vi "主界面.vi"() -> ()   [LabVIEW 2010]
uses:
  全局量/试验配置信息.vi
  全局量/全局_配置.vi
  全局量/自动测试结果.vi
panel:
  in  "进度提示":string
  in  "加载配置文件列表":u16(ring)
  out "配置文件路径":path
  out "配置文件目录":path
  in  "通道及参数配置":bool
  in  "?":enum32{"板卡类型1", "板卡类型2"}(tab)
  in  "单选_数字量输入":bool
  in  "单选_数字量输出":bool
  in  "单选_DSP输入":bool
  in  "单选_CAN检测":bool
  in  "单选_LAN检测":bool
  in  "单选_R232检测":bool
  in  "btn_数字输出":bool
  in  "btn_DSP输入":bool
  in  "btn_CAN总线":bool
  in  "btn_LAN总线":bool
  in  "btn_R232_485总线":bool
  in  "btn_开始检测":bool
  in  "btn_数字输入":bool
  in  "单选_R485检测":bool
  in  "单选_AD输入":bool
  out "数字量输入检测":bool
  out "数字量输出检测":bool
  out "模拟量DSP输入检测":bool
  out "模拟量AD输入检测":bool
  out "CAN总线检测":bool
  out "LAN总线检测":bool
  out "RS232总线检测":bool
  out "RS485总线检测":bool
  in  "btn_自动开始检测类型2":bool
  in  "函数类型 4":bool caption="y =f4(A1sin(2*π*A2)x+A3)"
  in  "函数类型 3":bool caption="y =f3(x)"
  in  "函数类型 2":bool caption="y =f2(x,A1,A2,t)"
  in  "函数类型 1":bool caption="y =f1(A1*x+A2)"
  out "函数类型4检测":bool
  out "函数类型3检测":bool
  out "函数类型2检测":bool
  out "函数类型1检测":bool
  in  "单选_函数类型4":bool
  in  "单选_函数类型3":bool
  in  "单选_函数类型2":bool
  in  "单选_函数类型1":bool
  in  "进度每次增加数":dbl
  in  "btn_二维码识别":bool
  out "退出？":bool
  in  "btn_退出":bool
  in  "btn_报告管理":bool
  in  "str_测试地点":string
  in  "str_测试人员":string
  in  "str_测试编号":string
  in  "str_报告编号":string
  # "板卡综合测试装置"
  # "板 卡 测 试 信 息"
  # "试验报告编号："
  # "测试板卡编号："
  # "板卡类型："
  # "测试人员："
  # "测试地点："
  # "自动测试"
  # "分步测试"
  # "测试\n项\n目"
  # "分步测试"
  # "自动测试"
  # "测试\n项\n目"
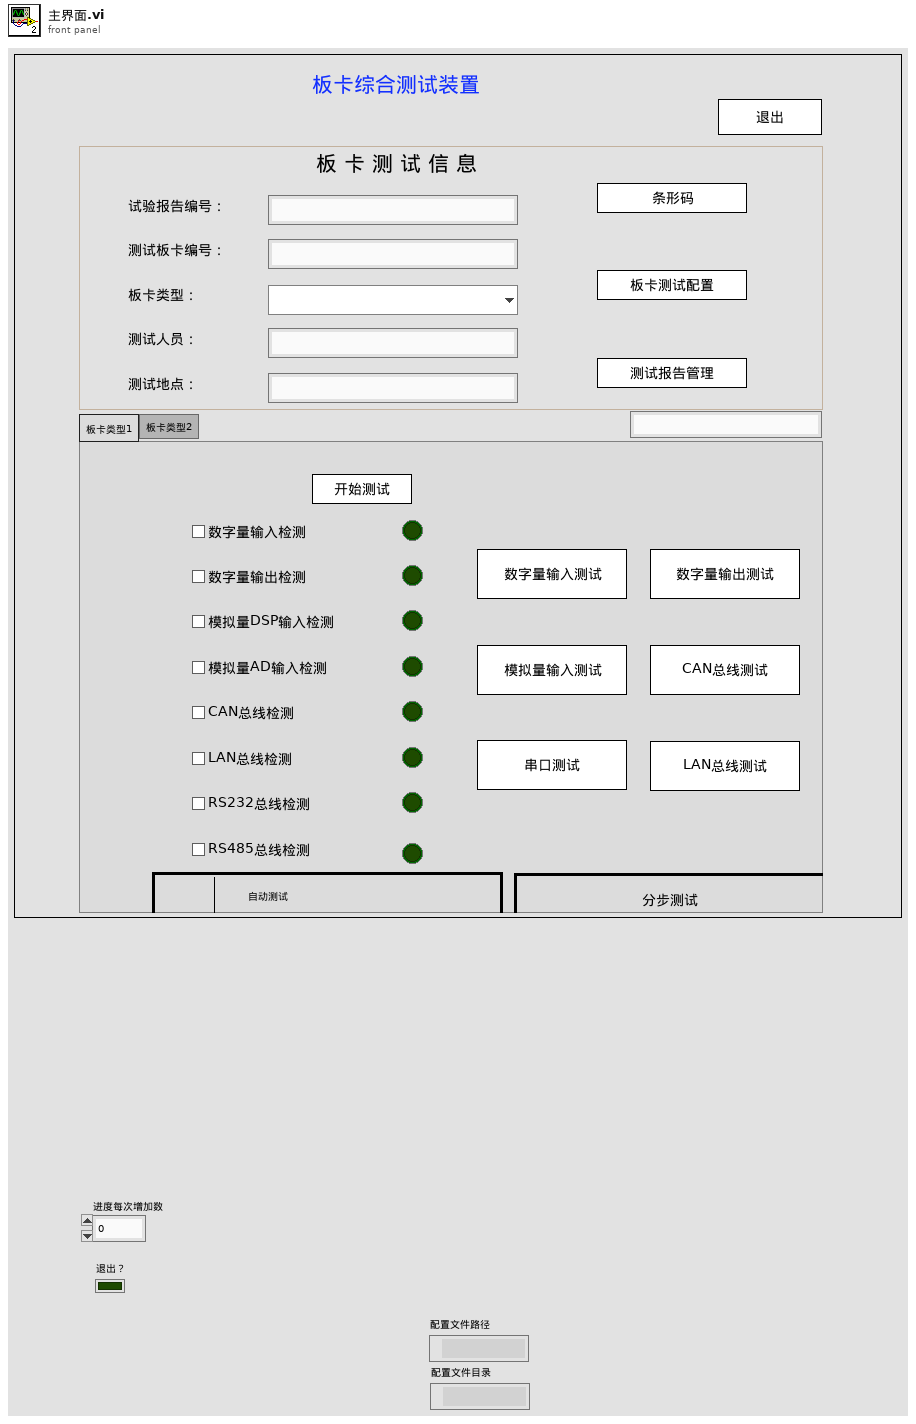
[diagram p1: front panel]
types:
  T1 = cluster{"str_报告编号":string, "str_测试编号":string, "RingText.Text":string, "str_测试人员":string, "str_测试地点":string}
  T2 = enum8{"Enabled", "Disabled", "Disabled and Grayed Out"}
  T3 = cluster{"数字量输入信号路数":i32, "数字量输出信号路数":i32, "DSP模拟量输入信号路数":u32, "DSP模拟量输入信号幅值":u32, "AD模拟量输入信号路数":u32, "AD模拟量输入信号幅值":u32, "RS232端口":u32, "RS232通信路数":u32, "RS232波特率":dbl, "RS485端口":u32, "RS485通信路数":u32, "RS485波特率":u32, "CAN通信路数":i32, "CAN波特率":u32, "以太网选择?":bool, "控制板IP":string, "以太网端口":u32}
  T4 = cluster{"str_报告编号":string, "str_测试编号":string, "RingText.Text":string, "str_测试地点":string, "str_测试人员":string}
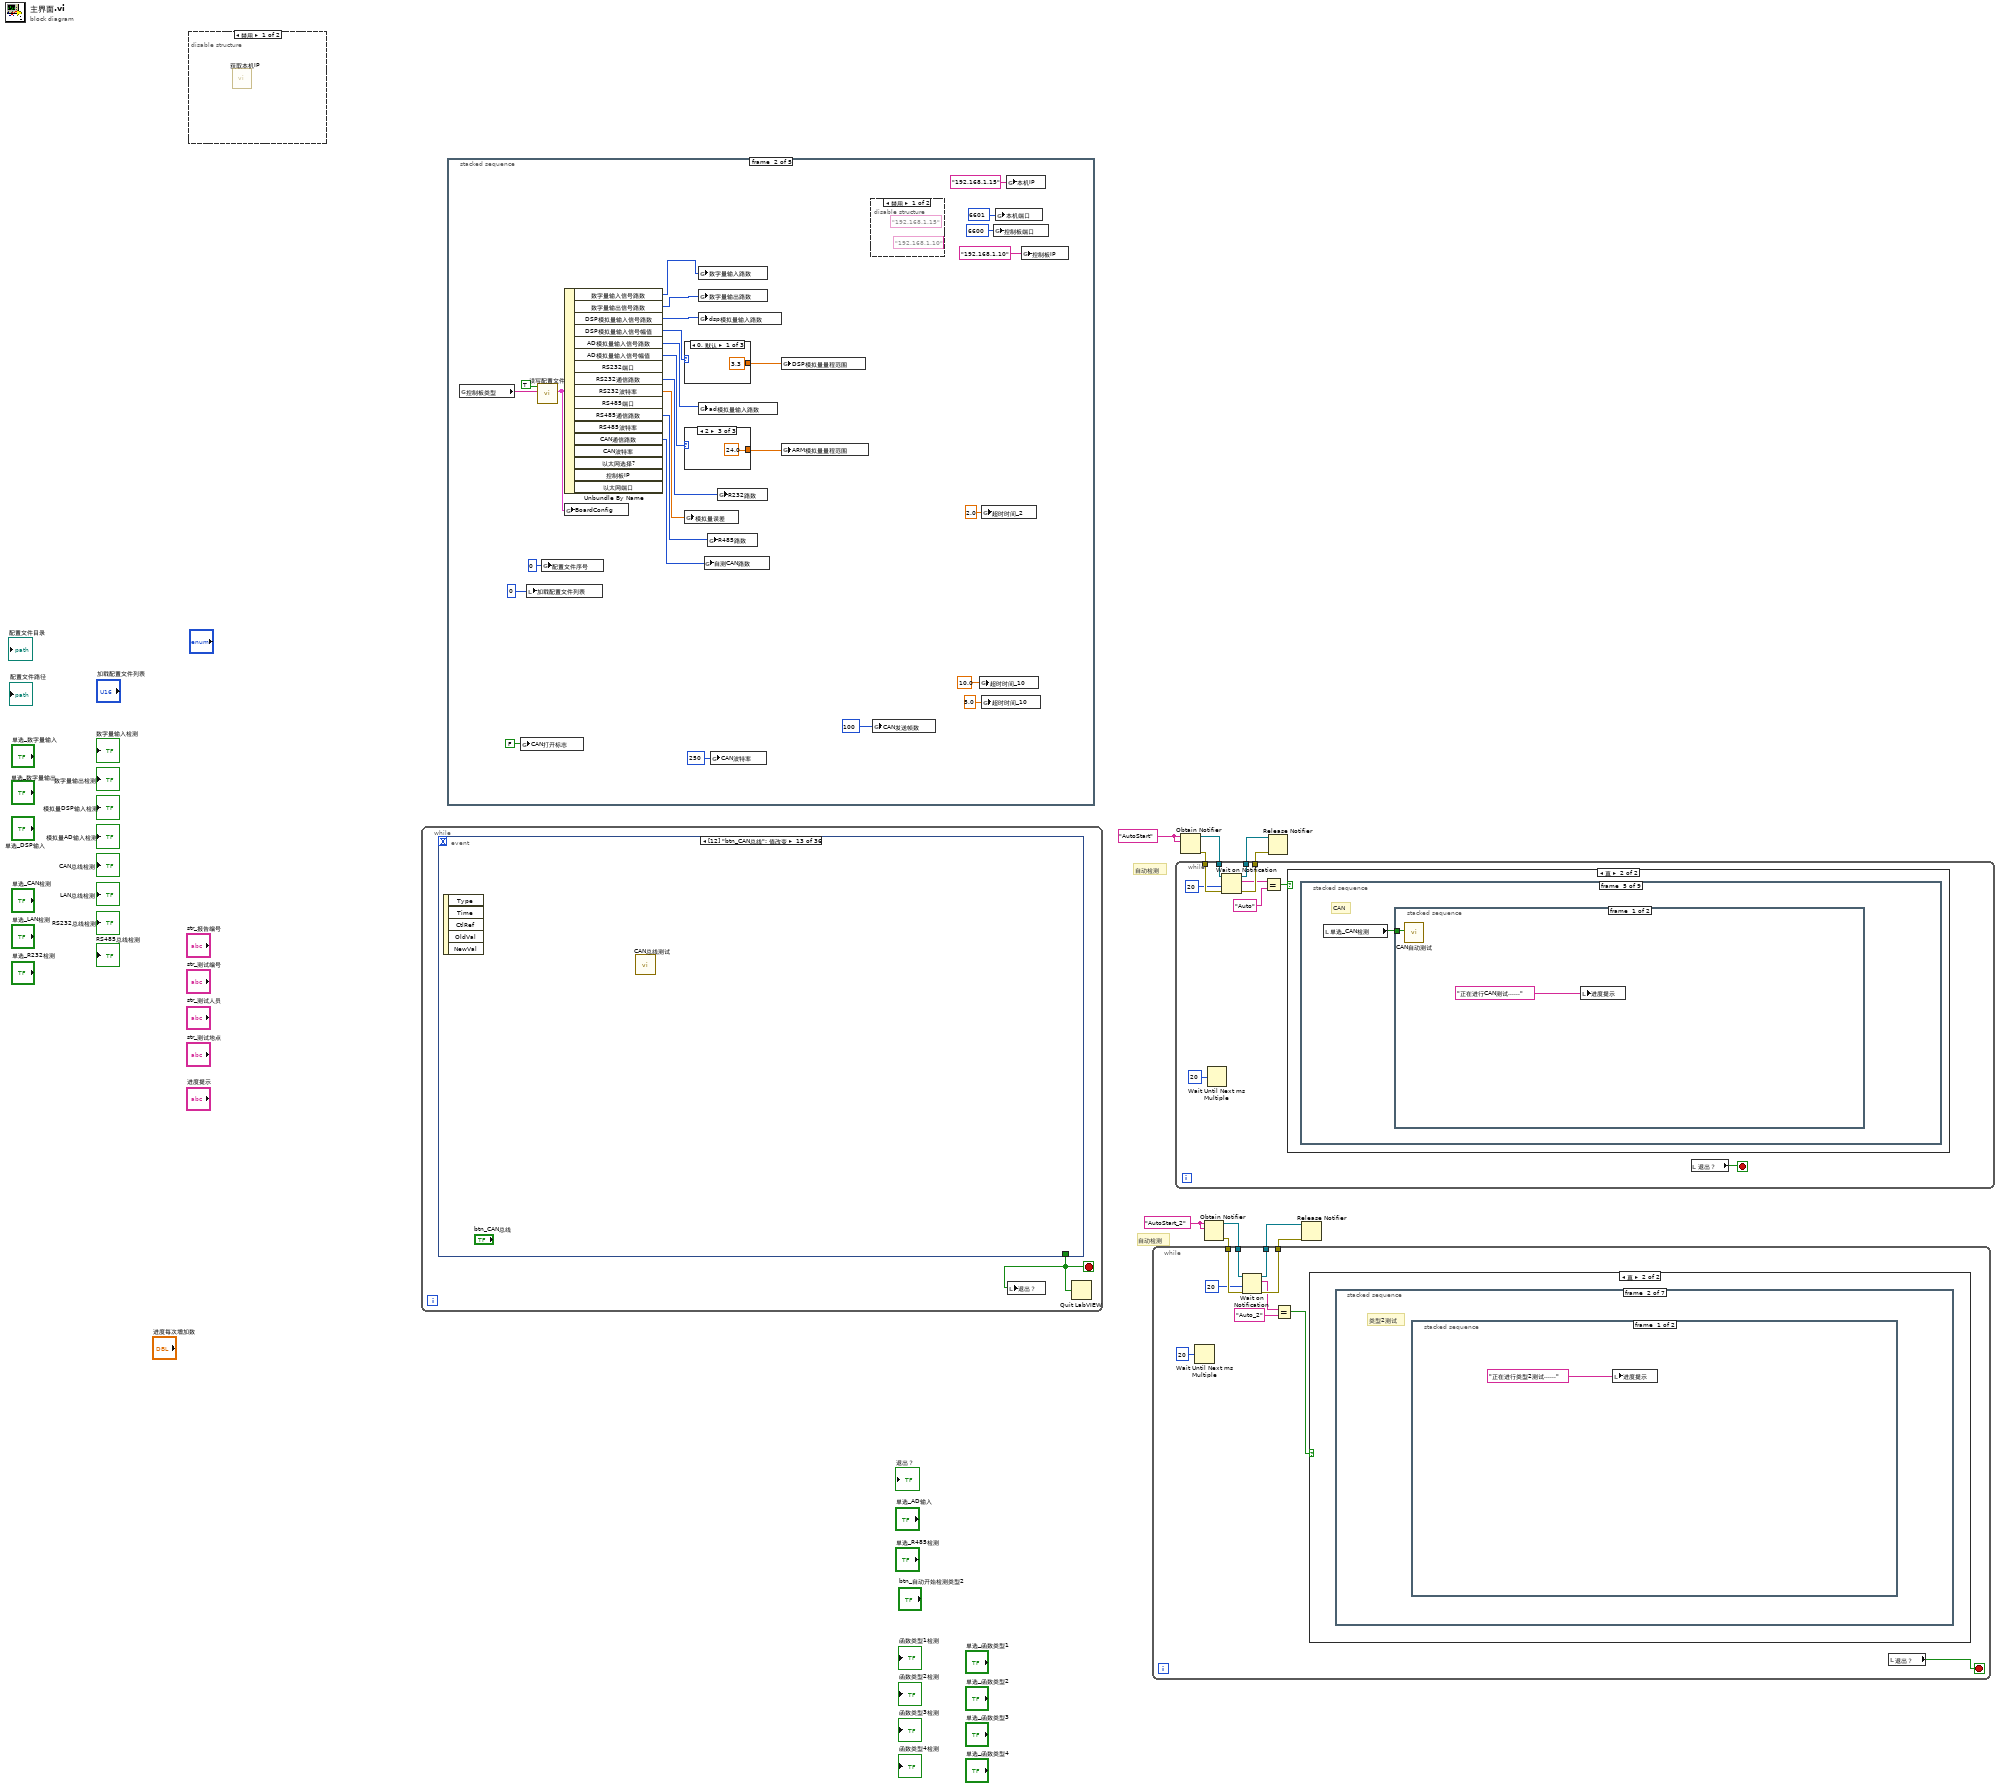
[diagram p0: block diagram]
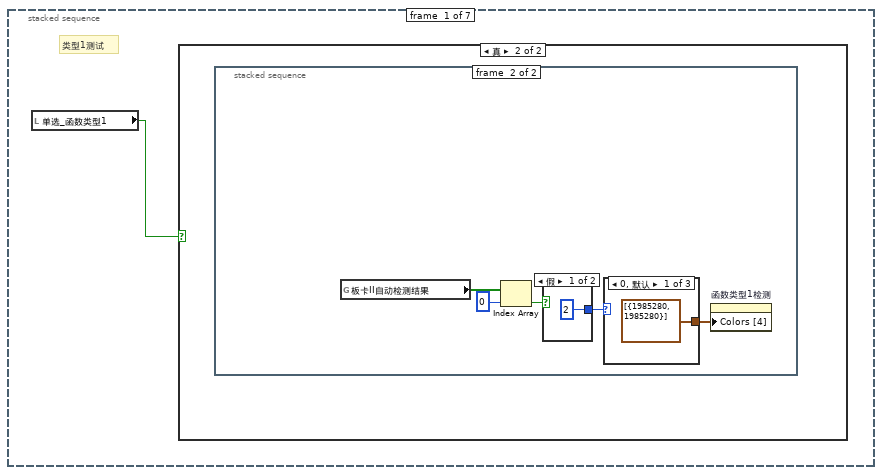
[diagram p4: hidden frame]
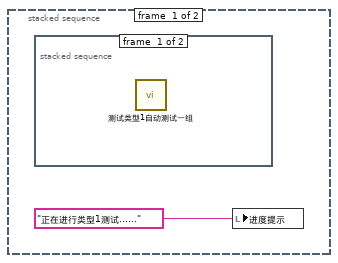
[diagram p6: hidden frame]
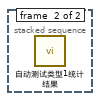
[diagram p7: hidden frame]
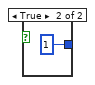
[diagram p8: hidden frame]
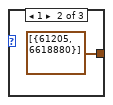
[diagram p9: hidden frame]
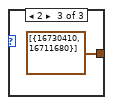
[diagram p10: hidden frame]
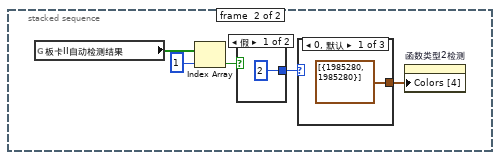
[diagram p11: hidden frame]
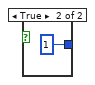
[diagram p12: hidden frame]
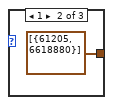
[diagram p13: hidden frame]
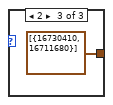
[diagram p14: hidden frame]
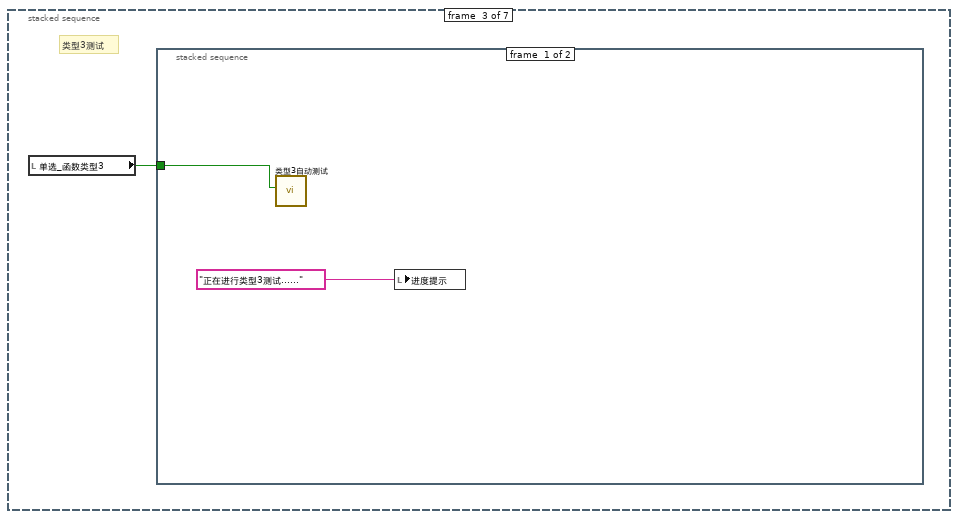
[diagram p15: hidden frame]
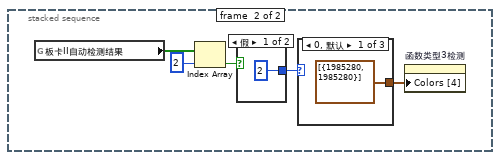
[diagram p16: hidden frame]
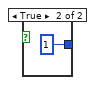
[diagram p17: hidden frame]
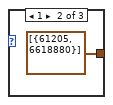
[diagram p18: hidden frame]
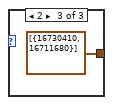
[diagram p19: hidden frame]
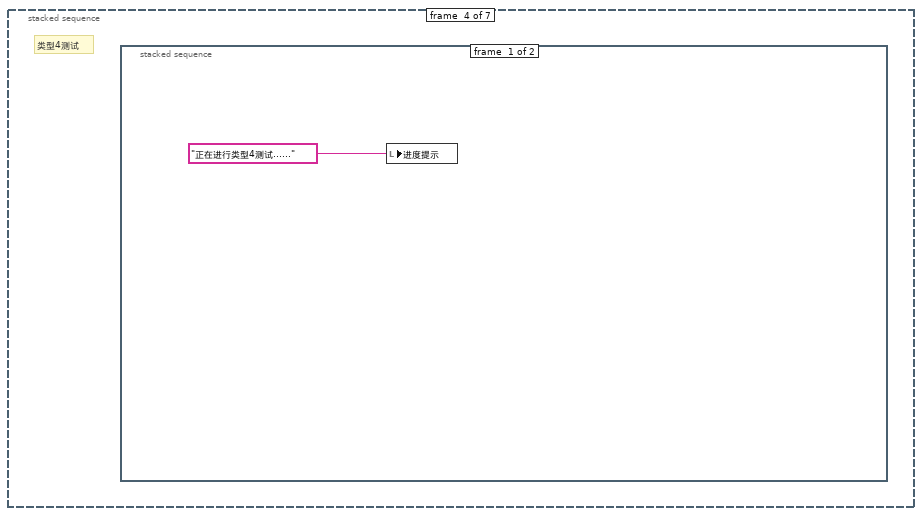
[diagram p20: hidden frame]
diagram:
  w5 = "AutoStart_2" ("名称（未命名）")
  w10 = "AutoStart" ("名称（未命名）")
  # "自动检测"
  # "自动检测"
  n1 = disable-structure shown="禁用" {
    frame Disabled {
      n2 = call "获取本机IP.vi"() -> ()  [unwired: 9 in, 3 out]
    }
    frame Enabled {
    }
  }
  n3 = while {
    stop <- w11 stop-if-true
    n4 = event shown="[12] \"btn_CAN总线\": 值改变" {
      selector: _ -> [_ _ _ _ _ _ _ _ _ _ _ _ _ _ _ _ _ _ _ _ _ _ _ _ _ _ _ _ _ _ _ _ _ _ _ _]
      dyn-events: _ -> [_ _ _ _ _ _ _ _ _ _ _ _ _ _ _ _ _ _ _ _ _ _ _ _ _ _ _ _ _ _ _ _ _ _ _ _]
      timeout: _ -> [_ _ _ _ _ _ _ _ _ _ _ _ _ _ _ _ _ _ _ _ _ _ _ _ _ _ _ _ _ _ _ _ _ _ _ _]
      tunnel: [_ w12 _ _ _ _ _ _ _ _ _ _ _ _ _ _ _ _ _ _ _ _ _ _ _ _ _ _ _ _ _ _ _ _ _ _] -> w11
      event Timeout {
        n5 = event-data() -> ()  [unwired: 1 in, 2 out]
      }
      event "btn_退出": Value Change {
        n6 = event-data() -> ()  [unwired: 1 in, 5 out]
        n7 = case shown="真" "btn_退出" {
          tunnel: [FALSE TRUE] -> w12
          frame False {
          }
          frame True {
          }
        }
      }
      event "btn_报告管理": Value Change {
        n8 = event-data() -> ()  [unwired: 1 in, 5 out]
        n9 = call "测试报告管理.vi"() -> ()  [unwired: 12 in]
      }
      event "单选_数字量输入": Value Change {
        n10 = event-data() -> ("NewVal"=w16:bool)  [unwired: 1 in, 4 out]
        n11 = local write "单选_数字量输入"(w16) -> ()
      }
      event "单选_数字量输出": Value Change {
        n12 = event-data() -> ("NewVal"=w17:bool)  [unwired: 1 in, 4 out]
        n13 = local write "单选_数字量输出"(w17) -> ()
      }
      event "单选_DSP输入": Value Change {
        n14 = event-data() -> ("NewVal"=w18:bool)  [unwired: 1 in, 4 out]
        n15 = local write "单选_DSP输入"(w18) -> ()
      }
      event "单选_CAN检测": Value Change {
        n16 = event-data() -> ("NewVal"=w19:bool)  [unwired: 1 in, 4 out]
        n17 = local write "单选_CAN检测"(w19) -> ()
      }
      event "单选_LAN检测": Value Change {
        n18 = event-data() -> ("NewVal"=w20:bool)  [unwired: 1 in, 4 out]
        n19 = local write "单选_LAN检测"(w20) -> ()
      }
      event "单选_R232检测": Value Change {
        n20 = event-data() -> ("NewVal"=w21:bool)  [unwired: 1 in, 4 out]
        n21 = local write "单选_R232检测"(w21) -> ()
      }
      event "btn_数字输入": Value Change {
        n22 = event-data() -> ()  [unwired: 1 in, 5 out]
        n23 = call "数字量输入配置.vi"() -> ()  [unwired: 12 in]
      }
      event "btn_数字输出": Value Change {
        n24 = event-data() -> ()  [unwired: 1 in, 5 out]
        n25 = call "数字量输出配置.vi"() -> ()  [unwired: 12 in]
      }
      event "btn_DSP输入": Value Change {
        n26 = event-data() -> ()  [unwired: 1 in, 5 out]
        n27 = call "32路模拟量输入.vi"() -> ()  [unwired: 12 in]
      }
      event "btn_CAN总线": Value Change {
        n28 = event-data() -> ()  [unwired: 1 in, 5 out]
        n29 = call "CAN总线测试.vi"() -> ()  [unwired: 12 in]
      }
      event "btn_LAN总线": Value Change {
        n30 = event-data() -> ()  [unwired: 1 in, 5 out]
        n31 = call "以太网测试界面.vi"() -> ()  [unwired: 12 in]
      }
      event "btn_R232_485总线": Value Change {
        n32 = event-data() -> ()  [unwired: 1 in, 5 out]
        n33 = call "RS232 485发送接收.vi"() -> ()  [unwired: 12 in]
      }
      event "btn_开始检测": Value Change {
        w23 = ""
        n34 = event-data() -> ()  [unwired: 1 in, 5 out]
        n35 = local read "单选_数字量输入"() -> (w32:bool)
        n36 = local read "单选_数字量输出"() -> (w31:bool)
        n37 = local read "单选_R232检测"() -> (w27:bool)
        n38 = local read "单选_R485检测"() -> (w28:bool)
        n39 = local read "单选_CAN检测"() -> (w25:bool)
        n40 = local read "单选_LAN检测"() -> (w26:bool)
        n41 = local read "单选_DSP输入"() -> (w30:bool)
        n42 = local read "单选_AD输入"() -> (w29:bool)
        n43 = local read "str_报告编号"() -> (w43:string)
        n44 = local read "str_测试编号"() -> (w42:string)
        n45 = local read "str_测试地点"() -> (w41:string)
        n46 = local read "str_测试人员"() -> (w40:string)
        n47 = property on="加载配置文件列表" class="Ring (严格)"() -> ("RingText.Text"=w24:string)  [unwired: 2 in, 2 out]
        n48 = Not Equal?(x=w43, y=w23) -> (x != y?=w39:bool)
        n49 = Not Equal?(x=w42, y=w23) -> (x != y?=w38:bool)
        n50 = Not Equal?(x=w41, y=w23) -> (x != y?=w37:bool)
        n51 = Not Equal?(x=w40, y=w23) -> (x != y?=w36:bool)
        n52 = Not Equal?(x=w24, y=w23) -> (x != y?=w22:bool)
        n53 = global write "试验配置信息.vi" "数字量输出选择？"(w31) -> ()
        n54 = global write "试验配置信息.vi" "数字量输入选择？"(w32) -> ()
        n55 = Compound Arithmetic op=AND(w22, w39, w38, w37, w36) -> (w34:bool)
        n56 = global write "试验配置信息.vi" "DSP输入选择？"(w30) -> ()
        n57 = global write "试验配置信息.vi" "CAN选择？"(w25) -> ()
        n58 = global write "试验配置信息.vi" "LAN选择？"(w26) -> ()
        n59 = global write "试验配置信息.vi" "RS232选择？"(w27) -> ()
        n60 = global write "试验配置信息.vi" "RS485选择？"(w28) -> ()
        n61 = global write "试验配置信息.vi" "AD输入选择？"(w29) -> ()
        n62 = Compound Arithmetic op=OR(w32, w31, w30, w25, w26, w27, w28, w29) -> (w33:bool)
        n63 = And(x=w34, y=w33) -> (x .and. y?=w35:bool)
        n64 = case shown="真" w35 {
          tunnel: w34 -> [w45 _]
          tunnel: w33 -> [w44 _]
          frame False {
            n65 = case shown="假" w44 {
              frame False {
                n66 = call "显示对话框信息2"() -> ()  [unwired: 10 in, 2 out]
              }
              frame True {
              }
            }
            n67 = case shown="假" w45 {
              frame False {
                n68 = call "显示对话框信息"() -> ()  [unwired: 10 in, 2 out]
              }
              frame True {
              }
            }
          }
          frame True {
            n69 = stacked-sequence {
              frame #0 {
                n70 = property on="加载配置文件列表" class="Ring (严格)"() -> ("RingText.Text"=w47:string)  [unwired: 2 in, 2 out]
                n71 = local read "str_报告编号"() -> (w53:string)
                n72 = local read "str_测试编号"() -> (w54:string)
                n73 = local read "str_测试地点"() -> (w56:string)
                n74 = local read "str_测试人员"() -> (w55:string)
                n75 = local read "str_测试地点"() -> (w46:string)
                n76 = local read "str_报告编号"() -> (w51:string)
                n77 = local read "str_测试编号"() -> (w50:string)
                n78 = local read "str_测试人员"() -> (w48:string)
                n79 = global write "试验配置信息.vi" "报告编号"(w53) -> ()
                n80 = global write "试验配置信息.vi" "控制板编号"(w54) -> ()
                n81 = global write "试验配置信息.vi" "测试地点"(w56) -> ()
                n82 = global write "试验配置信息.vi" "测试人员"(w55) -> ()
                n83 = Bundle("str_报告编号"=w51, "str_测试编号"=w50, "RingText.Text"=w47, "str_测试人员"=w48, "str_测试地点"=w46) -> (w49:T1)  [unwired: 1 in]
                n84 = global write "试验配置信息.vi" "控制板类型"(w47) -> ()
                n85 = call "实验配置信息读取和写入.vi"("读取写入"=TRUE, "输入簇"=w49) -> ()  [unwired: 7 in, 1 out]
              }
              frame #1 {
                n86 = local read "单选_数字量输入"() -> (w65:bool)
                n87 = local read "单选_数字量输出"() -> (w64:bool)
                n88 = local read "单选_R232检测"() -> (w59:bool)
                n89 = local read "单选_R485检测"() -> (w58:bool)
                n90 = local read "单选_CAN检测"() -> (w61:bool)
                n91 = local read "单选_LAN检测"() -> (w60:bool)
                n92 = local read "单选_DSP输入"() -> (w63:bool)
                n93 = local read "单选_AD输入"() -> (w57:bool)
                n94 = Build Array(w65, w64, w63, w61, w60, w59, w58, w57) -> (w62:bool[])
                n95 = for {
                  tunnel: w62 -> [w66] mode=indexing
                  n96 = case shown="真" w66 {
                    frame False {
                    }
                    frame True {
                      n97 = global read "试验配置信息.vi" "自测类数"() -> (w68:i32)
                      n98 = Increment(x=w68) -> (x+1=w67:i32)
                      n99 = global write "试验配置信息.vi" "自测类数"(w67) -> ()
                    }
                  }
                }
              }
              frame #2 {
                n100 = global read "试验配置信息.vi" "数字量输出选择？"() -> (w75:bool)
                n101 = global read "试验配置信息.vi" "数字量输入选择？"() -> (w76:bool)
                n102 = global read "试验配置信息.vi" "AD输入选择？"() -> (w73:bool)
                n103 = global read "试验配置信息.vi" "DSP输入选择？"() -> (w74:bool)
                n104 = global read "试验配置信息.vi" "CAN选择？"() -> (w72:bool)
                n105 = global read "试验配置信息.vi" "RS232选择？"() -> (w70:bool)
                n106 = global read "试验配置信息.vi" "RS485选择？"() -> (w69:bool)
                n107 = global read "试验配置信息.vi" "LAN选择？"() -> (w71:bool)
                n108 = case shown="真" w74 {
                  tunnel: [0 w95] -> w82
                  frame False {
                  }
                  frame True {
                    n109 = global read "全局_配置.vi" "dsp模拟量输入路数"() -> (w95:u32)
                  }
                }
                n110 = case shown="真" w73 {
                  tunnel: [0 w97] -> w83
                  frame False {
                  }
                  frame True {
                    n111 = global read "全局_配置.vi" "ad模拟量输入路数"() -> (w97:u32)
                  }
                }
                n112 = case shown="真" w75 {
                  tunnel: [0 w99] -> w84
                  frame False {
                  }
                  frame True {
                    n113 = global read "全局_配置.vi" "数字量输出路数"() -> (w99:i32)
                  }
                }
                n114 = case shown="真" w76 {
                  tunnel: [0 w101] -> w85
                  frame False {
                  }
                  frame True {
                    n115 = global read "全局_配置.vi" "数字量输入路数"() -> (w101:i32)
                  }
                }
                n116 = case shown="真" w72 {
                  tunnel: [0 w93] -> w81
                  frame False {
                  }
                  frame True {
                    n117 = global read "试验配置信息.vi" "自测CAN路数"() -> (w93:i32)
                  }
                }
                n118 = case shown="真" w70 {
                  tunnel: [0 w91] -> w80
                  frame False {
                  }
                  frame True {
                    n119 = global read "全局_配置.vi" "R232路数"() -> (w91:u32)
                  }
                }
                n120 = case shown="真" w69 {
                  tunnel: [0 w89] -> w79
                  frame False {
                  }
                  frame True {
                    n121 = global read "试验配置信息.vi" "自测485路数"() -> (w89:i32)
                  }
                }
                n122 = case shown="真" w71 {
                  tunnel: [0 w87] -> w78
                  frame False {
                  }
                  frame True {
                    n123 = global read "试验配置信息.vi" "自测LAN路数"() -> (w87:i32)
                  }
                }
                n124 = Compound Arithmetic op=ADD(w85, w84, w83, w82, w81, w80, w79, w78) -> (w77:u32)
                n125 = global write "试验配置信息.vi" "自测项数"(w77) -> ()
              }
              frame #3 {
                w109 = string[][] [["序号", "检测内容", "测试结果"]] ("自动测试结果")
                n126 = global read "全局_配置.vi" "dsp模拟量输入路数"() -> (w102:u32)
                n127 = global read "全局_配置.vi" "ad模拟量输入路数"() -> (w103:u32)
                n128 = Initialize Array(0.0 ("元素"), w102) -> (w104:dbl[])
                n129 = Initialize Array(0.0 ("元素"), w103) -> (w106:dbl[])
                n130 = global write "自动测试结果.vi" "总线通信自测结果"(w109) -> ()
                n131 = global write "自动测试结果.vi" "DI自动测试结果"(w109) -> ()
                n132 = global write "自动测试结果.vi" "DO自动测试结果"(w109) -> ()
                n133 = global write "自动测试结果.vi" "Auto_DSP_max_WC"(w104) -> ()
                n134 = global write "自动测试结果.vi" "Auto_AD_max_WC"(w106) -> ()
                n135 = global write "自动测试结果.vi" "AI自动测试结果"(string[][] [["序号", "检测内容", "最大误差(%)", "测试结果"]] ("自动测试结果")) -> ()
              }
              frame #4 {
                n136 = global read "试验配置信息.vi" "自测CAN路数"() -> (w126:i32)
                n137 = global read "试验配置信息.vi" "自测485路数"() -> (w129:i32)
                n138 = Initialize Array(TRUE ("元素"), w126) -> (w127:bool[])
                n139 = Initialize Array(TRUE ("元素"), w129) -> (w128:bool[])
                n140 = Initialize Array(TRUE ("元素"), 16 ("维数大小")) -> (w122:bool[])
                n141 = Initialize Array(TRUE ("元素"), 2 ("维数大小")) -> (w132:bool[])
                n142 = Initialize Array(TRUE ("元素"), 16 ("维数大小")) -> (w124:bool[])
                n143 = Initialize Array(TRUE, 5 ("维数大小"), 16 ("维数大小")) -> (w116:bool[][])
                n144 = Initialize Array(TRUE, 5 ("维数大小"), 16 ("维数大小")) -> (w120:bool[][])
                n145 = global write "自动测试结果.vi" "Auto_RS485_R"(w128) -> ()
                n146 = global write "自动测试结果.vi" "Auto_RS232_R"(w132) -> ()
                n147 = global write "自动测试结果.vi" "Auto_CAN_R"(w127) -> ()
                n148 = global write "自动测试结果.vi" "Auto_DSP_R"(w122) -> ()
                n149 = global write "自动测试结果.vi" "Auto_AD_R"(w124) -> ()
                n150 = global write "自动测试结果.vi" "Auto_DI_R"(w116) -> ()
                n151 = global write "自动测试结果.vi" "Auto_DO_R"(w120) -> ()
              }
              frame #5 {
                w133 = ""
                n152 = global read "试验配置信息.vi" "自测类数"() -> (w140:i32)
                n153 = global read "试验配置信息.vi" "自测项数"() -> (w137:i32)
                n154 = global read "试验配置信息.vi" "自测类数"() -> (w138:i32)
                n155 = global write "自动测试结果.vi" "数字量输入概述"(w133) -> ()
                n156 = global write "自动测试结果.vi" "数字量输出概述"(w133) -> ()
                n157 = global write "自动测试结果.vi" "模拟量DSP概述"(w133) -> ()
                n158 = global write "自动测试结果.vi" "模拟量AD概述结果"(w133) -> ()
                n159 = global write "自动测试结果.vi" "串口RS232测试概述"(w133) -> ()
                n160 = global write "自动测试结果.vi" "串口RS485测试概述"(w133) -> ()
                n161 = global write "自动测试结果.vi" "CAN测试概述"(w133) -> ()
                n162 = global write "自动测试结果.vi" "CAN测试概述"(w133) -> ()
                n163 = global write "自动测试结果.vi" "以太网测试概述"(w133) -> ()
                n164 = Divide(x=100, y=w140) -> (x/y=w142:dbl)
                n165 = property on="进度每次增加数" class="DigNum (严格)"("Value"=w142) -> ()  [unwired: 2 in, 2 out]
                n166 = Format Into String(format string="本报告测试项目共%d类，测试项总计%d项，其中：" ("时间格式字符串(%c)"), w138, w137) -> (resulting string=w135:string)  [unwired: 2 in, 1 out]
                n167 = Concatenate Strings(w135, "\r") -> (w136:string)
                n168 = global write "自动测试结果.vi" "自测总概述"(w136) -> ()
              }
              frame #6 {
                w145 = "AutoStart" ("名称（未命名）")
                n169 = Obtain Notifier(name (unnamed)=w145, notification data type=w145) -> (notifier out=w144:refnum<notifier>)  [unwired: 2 in, 2 out]
                n170 = local write "进度提示"("正在测试中，请耐心等待结果......") -> ()
                n171 = Send Notification(notification="Auto" ("通知"), notifier=w144) -> ()  [unwired: 1 in, 2 out]
              }
              frame #7 {
                w147 = T2."Disabled and Grayed Out" ("禁用")
                n172 = property on="btn_数字输入" class="Bool"("DisabledEnum"=w147) -> ()  [unwired: 2 in, 2 out]
                n173 = property on="btn_数字输出" class="Bool"("DisabledEnum"=w147) -> ()  [unwired: 2 in, 2 out]
                n174 = property on="btn_DSP输入" class="Bool"("DisabledEnum"=w147) -> ()  [unwired: 2 in, 2 out]
                n175 = property on="btn_CAN总线" class="Bool"("DisabledEnum"=w147) -> ()  [unwired: 2 in, 2 out]
                n176 = property on="btn_R232_485总线" class="Bool"("DisabledEnum"=w147) -> ()  [unwired: 2 in, 2 out]
                n177 = property on="btn_LAN总线" class="Bool"("DisabledEnum"=w147) -> ()  [unwired: 2 in, 2 out]
                n178 = property on="函数类型 1" class="Bool"("DisabledEnum"=w147) -> ()  [unwired: 2 in, 2 out]
                n179 = property on="函数类型 2" class="Bool"("DisabledEnum"=w147) -> ()  [unwired: 2 in, 2 out]
                n180 = property on="函数类型 3" class="Bool"("DisabledEnum"=w147) -> ()  [unwired: 2 in, 2 out]
                n181 = property on="函数类型 4" class="Bool"("DisabledEnum"=w147) -> ()  [unwired: 2 in, 2 out]
                n182 = property on="btn_自动开始检测类型2" class="Bool"("DisabledEnum"=w147) -> ()  [unwired: 2 in, 2 out]
              }
            }
          }
        }
      }
      event "加载配置文件列表": Value Change {
        n183 = event-data() -> ()  [unwired: 1 in, 5 out]
        n184 = stacked-sequence {
          frame #0 {
            n185 = property on="加载配置文件列表" class="Ring (严格)"() -> ("RingText.Text"=w148:string)  [unwired: 2 in, 2 out]
            n186 = global write "试验配置信息.vi" "控制板类型"(w148) -> ()
          }
          frame #1 {
            # "待读取配置文件路径"
            n187 = local read "配置文件目录"() -> (w149:path)
            n188 = global read "试验配置信息.vi" "控制板类型"() -> (w151:string)
            n189 = Build Path(base path=w149, name or relative path=w151) -> (appended path=w150:path)
            n190 = local write "配置文件路径"(w150) -> ()
          }
          frame #2 {
            n191 = local read "配置文件路径"() -> (w152:path)
            n192 = call "函数测试配置文件读取.vi"("配置文件路径"=w152) -> ("D_IN_4"=w156:string[][], "D_IN_3"=w155:string[][], "D_IN_2"=w154:string[][], "D_IN_1"=w153:string[][])  [unwired: 6 in]
            n193 = global write "试验配置信息.vi" "D_IN_1"(w153) -> ()
            n194 = global write "试验配置信息.vi" "D_IN_2"(w154) -> ()
            n195 = global write "试验配置信息.vi" "D_IN_3"(w155) -> ()
            n196 = global write "试验配置信息.vi" "D_IN_4"(w156) -> ()
          }
          frame #3 {
            n197 = global read "试验配置信息.vi" "控制板类型"() -> (w165:string)
            n198 = call "读写配置文件.vi"("文件名称"=w165, "m_bRead"=TRUE) -> ("BoardConfig_output"=w166:T3)  [unwired: 9 in]
            n199 = global write "全局_配置.vi" "BoardConfig"(w166) -> ()
            n200 = Unbundle By Name(w166) -> ("数字量输入信号路数"=w163:i32, "数字量输出信号路数"=w162:i32, "DSP模拟量输入信号路数"=w161:u32, "DSP模拟量输入信号幅值"=w168:u32, "AD模拟量输入信号路数"=w160:u32, "AD模拟量输入信号幅值"=w171:u32, "RS232通信路数"=w159:u32, "RS232波特率"=w167:dbl, "RS485通信路数"=w158:u32, "CAN通信路数"=w157:i32)  [unwired: 7 out]
            n201 = case shown="0, 默认" w168 {
              tunnel: [3.3 10.0 24.0] -> w169
              frame 0, Default {
              }
              frame 1 {
              }
              frame 2 {
              }
            }
            n202 = case shown="2" w171 {
              tunnel: [6.0 10.0 24.0] -> w170
              frame 0, Default {
              }
              frame 1 {
              }
              frame 2 {
              }
            }
            n203 = global write "全局_配置.vi" "模拟量误差"(w167) -> ()
            n204 = global write "全局_配置.vi" "dsp模拟量输入路数"(w161) -> ()
            n205 = global write "全局_配置.vi" "数字量输出路数"(w162) -> ()
            n206 = global write "全局_配置.vi" "数字量输入路数"(w163) -> ()
            n207 = global write "全局_配置.vi" "ad模拟量输入路数"(w160) -> ()
            n208 = global write "试验配置信息.vi" "自测CAN路数"(w157) -> ()
            n209 = global write "全局_配置.vi" "R485路数"(w158) -> ()
            n210 = global write "全局_配置.vi" "R232路数"(w159) -> ()
            n211 = global write "全局_配置.vi" "DSP模拟量量程范围"(w169) -> ()
            n212 = global write "全局_配置.vi" "ARM模拟量量程范围"(w170) -> ()
          }
        }
      }
      event "btn_自动开始检测类型2": Value Change {
        n213 = event-data() -> ()  [unwired: 1 in, 5 out]
        n214 = local read "单选_函数类型1"() -> (w185:bool)
        n215 = local read "单选_函数类型2"() -> (w184:bool)
        n216 = local read "单选_函数类型3"() -> (w183:bool)
        n217 = local read "单选_函数类型4"() -> (w182:bool)
        n218 = local read "str_报告编号"() -> (w193:string)
        n219 = local read "str_测试编号"() -> (w192:string)
        n220 = local read "str_测试地点"() -> (w191:string)
        n221 = local read "str_测试人员"() -> (w190:string)
        n222 = property on="加载配置文件列表" class="Ring (严格)"() -> ("RingText.Text"=w178:string)  [unwired: 2 in, 2 out]
        n223 = Not Equal?(x=w193, y=w178) -> (x != y?=w189:bool)
        n224 = Not Equal?(x=w192, y=w178) -> (x != y?=w188:bool)
        n225 = Not Equal?(x=w191, y=w178) -> (x != y?=w187:bool)
        n226 = Not Equal?(x=w190, y=w178) -> (x != y?=w186:bool)
        n227 = global write "试验配置信息.vi" "测试类型1选择？"(w185) -> ()
        n228 = global write "试验配置信息.vi" "测试类型2选择？"(w184) -> ()
        n229 = global write "试验配置信息.vi" "测试类型3选择？"(w183) -> ()
        n230 = global write "试验配置信息.vi" "测试类型4选择？"(w182) -> ()
        n231 = Compound Arithmetic op=AND(w189, w188, w187, w186) -> (w180:bool)
        n232 = Compound Arithmetic op=OR(w185, w184, w183, w182) -> (w179:bool)
        n233 = And(x=w180, y=w179) -> (x .and. y?=w181:bool)
        n234 = case shown="真" w181 {
          tunnel: w180 -> [w195 _]
          tunnel: w179 -> [w194 _]
          frame False {
            n235 = case shown="假" w195 {
              frame False {
                n236 = call "显示对话框信息3"() -> ()  [unwired: 10 in, 2 out]
              }
              frame True {
              }
            }
            n237 = case shown="假" w194 {
              frame False {
                n238 = call "显示对话框信息4"() -> ()  [unwired: 10 in, 2 out]
              }
              frame True {
              }
            }
          }
          frame True {
            n239 = stacked-sequence {
              frame #0 {
                n240 = property on="加载配置文件列表" class="Ring (严格)"() -> ("RingText.Text"=w199:string)  [unwired: 2 in, 2 out]
                n241 = local read "str_报告编号"() -> (w203:string)
                n242 = local read "str_测试编号"() -> (w204:string)
                n243 = local read "str_测试地点"() -> (w206:string)
                n244 = local read "str_测试人员"() -> (w205:string)
                n245 = local read "str_报告编号"() -> (w201:string)
                n246 = local read "str_测试编号"() -> (w200:string)
                n247 = local read "str_测试地点"() -> (w198:string)
                n248 = local read "str_测试人员"() -> (w197:string)
                n249 = global write "试验配置信息.vi" "报告编号"(w203) -> ()
                n250 = global write "试验配置信息.vi" "控制板编号"(w204) -> ()
                n251 = global write "试验配置信息.vi" "测试地点"(w206) -> ()
                n252 = global write "试验配置信息.vi" "测试人员"(w205) -> ()
                n253 = Bundle("str_报告编号"=w201, "str_测试编号"=w200, "RingText.Text"=w199, "str_测试地点"=w198, "str_测试人员"=w197) -> (w196:T4)  [unwired: 1 in]
                n254 = global write "试验配置信息.vi" "控制板类型"(w199) -> ()
                n255 = call "实验配置信息读取和写入.vi"("读取写入"=TRUE, "输入簇"=w196) -> ()  [unwired: 7 in, 1 out]
              }
              frame #1 {
                n256 = local read "单选_函数类型1"() -> (w211:bool)
                n257 = local read "单选_函数类型2"() -> (w210:bool)
                n258 = local read "单选_函数类型3"() -> (w209:bool)
                n259 = local read "单选_函数类型4"() -> (w208:bool)
                n260 = Build Array(w211, w210, w209, w208) -> (w207:bool[])
                n261 = for {
                  tunnel: w207 -> [w212] mode=indexing
                  n262 = case shown="真" w212 {
                    frame False {
                    }
                    frame True {
                      n263 = global read "试验配置信息.vi" "自测类数"() -> (w214:i32)
                      n264 = Increment(x=w214) -> (x+1=w213:i32)
                      n265 = global write "试验配置信息.vi" "自测类数"(w213) -> ()
                    }
                  }
                }
              }
              frame #2 {
                n266 = global read "试验配置信息.vi" "测试类型1选择？"() -> (w223:bool)
                n267 = global read "试验配置信息.vi" "测试类型2选择？"() -> (w222:bool)
                n268 = global read "试验配置信息.vi" "测试类型3选择？"() -> (w221:bool)
                n269 = global read "试验配置信息.vi" "测试类型4选择？"() -> (w220:bool)
                n270 = case shown="真" w223 {
                  tunnel: [0 w231] -> w219
                  frame False {
                  }
                  frame True {
                    n271 = global read "试验配置信息.vi" "自测类型1路数"() -> (w231:i32)
                  }
                }
                n272 = case shown="真" w221 {
                  tunnel: [0 w227] -> w217
                  frame False {
                  }
                  frame True {
                    n273 = global read "试验配置信息.vi" "自测类型3路数"() -> (w227:i32)
                  }
                }
                n274 = case shown="真" w222 {
                  tunnel: [0 w229] -> w218
                  frame False {
                  }
                  frame True {
                    n275 = global read "试验配置信息.vi" "自测类型2路数"() -> (w229:i32)
                  }
                }
                n276 = case shown="真" w220 {
                  tunnel: [0 w225] -> w216
                  frame False {
                  }
                  frame True {
                    n277 = global read "试验配置信息.vi" "自测类型4路数"() -> (w225:i32)
                  }
                }
                n278 = Compound Arithmetic op=ADD(w219, w218, w217, w216) -> (w215:i32)
                n279 = global write "试验配置信息.vi" "自测项数"(w215) -> ()
              }
              frame #3 {
                n280 = global read "试验配置信息.vi" "自测类型1路数"() -> (w236:i32)
                n281 = global read "试验配置信息.vi" "自测类型2路数"() -> (w239:i32)
                n282 = global read "试验配置信息.vi" "自测类型3路数"() -> (w242:i32)
                n283 = global read "试验配置信息.vi" "自测类型4路数"() -> (w245:i32)
                n284 = global read "试验配置信息.vi" "自测类型1路数"() -> (w232:i32)
                n285 = Initialize Array(TRUE ("元素"), w236) -> (w235:bool[])
                n286 = Initialize Array(TRUE ("元素"), w239) -> (w240:bool[])
                n287 = Initialize Array(TRUE ("元素"), w242) -> (w241:bool[])
                n288 = Initialize Array(TRUE ("元素"), w245) -> (w246:bool[])
                n289 = Initialize Array(0.0, w232) -> (w234:dbl[])
                n290 = global write "自动测试结果.vi" "Auto_func_1_R"(w235) -> ()
                n291 = global write "自动测试结果.vi" "Auto_func_2_R"(w240) -> ()
                n292 = global write "自动测试结果.vi" "Auto_func_3_R"(w241) -> ()
                n293 = global write "自动测试结果.vi" "Auto_func_4_R"(w246) -> ()
                n294 = global write "自动测试结果.vi" "Auto_func_1_max_WC"(w234) -> ()
              }
              frame #4 {
                w247 = string[][] [["序号", "输出通道", "输入通道", "测试结果", ""]] ("自动测试结果")
                w249 = ""
                n295 = global read "试验配置信息.vi" "自测项数"() -> (w253:i32)
                n296 = global read "试验配置信息.vi" "自测类数"() -> (w254:i32)
                n297 = global write "自动测试结果.vi" "测试类型1概述"(w249) -> ()
                n298 = global write "自动测试结果.vi" "测试类型2概述"(w249) -> ()
                n299 = global write "自动测试结果.vi" "测试类型3概述"(w249) -> ()
                n300 = global write "自动测试结果.vi" "测试类型4概述"(w249) -> ()
                n301 = Format Into String(format string="本报告测试项目共%d类，测试项总计%d项，其中：" ("时间格式字符串(%c)"), w254, w253) -> (resulting string=w251:string)  [unwired: 2 in, 1 out]
                n302 = global write "自动测试结果.vi" "测试类型1自动测试结果"(string[][] [["序号", "输出通道", "输入通道试结果", "最大误差(%)", "测试结果"]] ("自动测试结果")) -> ()
                n303 = global write "自动测试结果.vi" "测试类型2自动测试结果"(w247) -> ()
                n304 = global write "自动测试结果.vi" "测试类型3自动测试结果"(w247) -> ()
                n305 = global write "自动测试结果.vi" "测试类型4自动测试结果"(w247) -> ()
                n306 = Concatenate Strings(w251, "\r") -> (w252:string)
                n307 = global write "自动测试结果.vi" "自测总概述"(w252) -> ()
              }
              frame #5 {
                w258 = "AutoStart_2" ("名称（未命名）")
                n308 = Obtain Notifier(name (unnamed)=w258, notification data type=w258) -> (notifier out=w257:refnum<notifier>)  [unwired: 2 in, 2 out]
                n309 = local write "进度提示"("正在测试中，请耐心等待结果......") -> ()
                n310 = Send Notification(notification="Auto_2" ("通知"), notifier=w257) -> ()  [unwired: 1 in, 2 out]
              }
              frame #6 {
                w260 = T2."Disabled and Grayed Out" ("禁用")
                n311 = property on="btn_数字输入" class="Bool"("DisabledEnum"=w260) -> ()  [unwired: 2 in, 2 out]
                n312 = property on="btn_数字输出" class="Bool"("DisabledEnum"=w260) -> ()  [unwired: 2 in, 2 out]
                n313 = property on="btn_DSP输入" class="Bool"("DisabledEnum"=w260) -> ()  [unwired: 2 in, 2 out]
                n314 = property on="btn_CAN总线" class="Bool"("DisabledEnum"=w260) -> ()  [unwired: 2 in, 2 out]
                n315 = property on="btn_R232_485总线" class="Bool"("DisabledEnum"=w260) -> ()  [unwired: 2 in, 2 out]
                n316 = property on="btn_LAN总线" class="Bool"("DisabledEnum"=w260) -> ()  [unwired: 2 in, 2 out]
                n317 = property on="函数类型 1" class="Bool"("DisabledEnum"=w260) -> ()  [unwired: 2 in, 2 out]
                n318 = property on="函数类型 2" class="Bool"("DisabledEnum"=w260) -> ()  [unwired: 2 in, 2 out]
                n319 = property on="函数类型 3" class="Bool"("DisabledEnum"=w260) -> ()  [unwired: 2 in, 2 out]
                n320 = property on="函数类型 4" class="Bool"("DisabledEnum"=w260) -> ()  [unwired: 2 in, 2 out]
                n321 = property on="btn_开始检测" class="Bool"("DisabledEnum"=w260) -> ()  [unwired: 2 in, 2 out]
              }
            }
          }
        }
      }
      event "单选_函数类型1": Value Change {
        n322 = event-data() -> ("NewVal"=w261:bool)  [unwired: 1 in, 4 out]
        n323 = local write "单选_函数类型1"(w261) -> ()
      }
      event "单选_函数类型2": Value Change {
        n324 = event-data() -> ("NewVal"=w262:bool)  [unwired: 1 in, 4 out]
        n325 = local write "单选_函数类型2"(w262) -> ()
      }
      event "单选_函数类型3": Value Change {
        n326 = event-data() -> ("NewVal"=w263:bool)  [unwired: 1 in, 4 out]
        n327 = local write "单选_函数类型3"(w263) -> ()
      }
      event "单选_函数类型4": Value Change {
        n328 = event-data() -> ("NewVal"=w264:bool)  [unwired: 1 in, 4 out]
        n329 = local write "单选_函数类型4"(w264) -> ()
      }
      event "通道及参数配置": Value Change {
        n330 = event-data() -> ()  [unwired: 1 in, 5 out]
        n331 = call "通道配置模块.vi"() -> ("返回"=w265:bool)  [unwired: 11 in]
        n332 = case shown="真" w265 {
          frame False {
          }
          frame True {
            n333 = global read "试验配置信息.vi" "配置文件序号"() -> (w266:u16)
            n334 = property on="加载配置文件列表" class="Ring (严格)"("Value"=w266) -> ()  [unwired: 2 in, 2 out]
          }
        }
      }
      event "btn_二维码识别": Value Change {
        n335 = event-data() -> ()  [unwired: 1 in, 5 out]
        n336 = call "生成板卡编号.vi"() -> ()  [unwired: 12 in]
      }
      event "函数类型 1": Value Change {
        n337 = event-data() -> ()  [unwired: 1 in, 5 out]
        n338 = call "函数类型1测试.vi"() -> ()  [unwired: 12 in]
      }
      event "函数类型 1": Mouse Leave {
        n339 = event-data() -> ()  [unwired: 1 in, 3 out]
        n340 = property on="函数类型 1" class="Bool"("Caption.Visible"=FALSE ("标签.可见")) -> ()  [unwired: 2 in, 2 out]
      }
      event "函数类型 1": Mouse Enter {
        n341 = event-data() -> ()  [unwired: 1 in, 3 out]
        n342 = property on="函数类型 1" class="Bool"("Caption.Visible"=TRUE ("标签.可见")) -> ()  [unwired: 2 in, 2 out]
      }
      event "函数类型 2": Value Change {
        n343 = event-data() -> ()  [unwired: 1 in, 5 out]
        n344 = call "函数类型2测试.vi"() -> ()  [unwired: 12 in]
      }
      event "函数类型 2": Mouse Enter {
        n345 = event-data() -> ()  [unwired: 1 in, 3 out]
        n346 = property on="函数类型 2" class="Bool"("Caption.Visible"=TRUE) -> ()  [unwired: 2 in, 2 out]
      }
      event "函数类型 2": Mouse Leave {
        n347 = event-data() -> ()  [unwired: 1 in, 3 out]
        n348 = property on="函数类型 2" class="Bool"("Caption.Visible"=FALSE) -> ()  [unwired: 2 in, 2 out]
      }
      event "函数类型 3": Value Change {
        n349 = event-data() -> ()  [unwired: 1 in, 5 out]
        n350 = call "函数类型3测试.vi"() -> ()  [unwired: 12 in]
      }
      event "函数类型 3": Mouse Enter {
        n351 = event-data() -> ()  [unwired: 1 in, 3 out]
        n352 = property on="函数类型 3" class="Bool"("Caption.Visible"=TRUE) -> ()  [unwired: 2 in, 2 out]
      }
      event "函数类型 3": Mouse Leave {
        n353 = event-data() -> ()  [unwired: 1 in, 3 out]
        n354 = property on="函数类型 3" class="Bool"("Caption.Visible"=FALSE) -> ()  [unwired: 2 in, 2 out]
      }
      event "函数类型 4": Value Change {
        n355 = event-data() -> ()  [unwired: 1 in, 5 out]
        n356 = call "函数类型4测试.vi"() -> ()  [unwired: 12 in]
      }
      event "函数类型 4": Mouse Enter {
        n357 = event-data() -> ()  [unwired: 1 in, 3 out]
        n358 = property on="函数类型 4" class="Bool"("Caption.Visible"=TRUE) -> ()  [unwired: 2 in, 2 out]
      }
      event "函数类型 4": Mouse Leave {
        n359 = event-data() -> ()  [unwired: 1 in, 3 out]
        n360 = property on="函数类型 4" class="Bool"("Caption.Visible"=FALSE) -> ()  [unwired: 2 in, 2 out]
      }
    }
    n361 = local write "退出？"(w11) -> ()
    n362 = Quit LabVIEW(quit? (T)=w11) -> ()
  }
  n363 = stacked-sequence {
    frame #0 {
      n364 = stacked-sequence {
        frame #0 {
          # "初始化配置文件路径"
          n365 = VI Library "VI库"() -> (path=w283:path)
          n366 = Strip Path(path=w283) -> (stripped path=w282:path)  [unwired: 1 out]
          n367 = Build Path(base path=w282, name or relative path="config" ("名称或相对路径")) -> (appended path=w280:path)
          n368 = Build Path(base path=w280, name or relative path="bordII_config" ("名称或相对路径")) -> (appended path=w276:path)
          n369 = call <vilib>:"Check if File or Folder Exists.vi"("path"=w276) -> ("file or folder exists?"=w277:bool, "dup path"=w278:path)  [unwired: 8 in, 1 out]
          n370 = case shown="假" w277 {
            tunnel: w278 -> [w284 w286]
            tunnel: [w285 w286] -> w275
            frame False {
              n371 = Create Folder(path (use dialog)=w284) -> (created path=w285:path)  [unwired: 2 in, 2 out]
            }
            frame True {
            }
          }
          n372 = local write "配置文件目录"(w275) -> ()
        }
        frame #1 {
          # "遍历配置文件目录"
          n373 = local read "配置文件目录"() -> (w288:path)
          n374 = call "罗列目录配置文件.vi"("路径"=w288) -> ("数组"=w287:string[])  [unwired: 10 in]
          n375 = property on="加载配置文件列表" class="Ring (严格)"("Strings []"=w287) -> ()  [unwired: 2 in, 2 out]
        }
        frame #2 {
          n376 = property on="加载配置文件列表" class="Ring (严格)"() -> ("RingText.Text"=w289:string)  [unwired: 2 in, 2 out]
          n377 = global write "试验配置信息.vi" "控制板类型"(w289) -> ()
        }
        frame #3 {
          # "待读取配置文件路径"
          n378 = local read "配置文件目录"() -> (w292:path)
          n379 = global read "试验配置信息.vi" "控制板类型"() -> (w290:string)
          n380 = Build Path(base path=w292, name or relative path=w290) -> (appended path=w291:path)
          n381 = local write "配置文件路径"(w291) -> ()
        }
        frame #4 {
          n382 = local read "配置文件路径"() -> (w297:path)
          n383 = call "函数测试配置文件读取.vi"("配置文件路径"=w297) -> ("D_IN_4"=w293:string[][], "D_IN_3"=w294:string[][], "D_IN_2"=w295:string[][], "D_IN_1"=w296:string[][])  [unwired: 6 in]
          n384 = global write "试验配置信息.vi" "D_IN_1"(w296) -> ()
          n385 = global write "试验配置信息.vi" "D_IN_2"(w295) -> ()
          n386 = global write "试验配置信息.vi" "D_IN_3"(w294) -> ()
          n387 = global write "试验配置信息.vi" "D_IN_4"(w293) -> ()
        }
      }
    }
    frame #1 {
      n388 = global read "试验配置信息.vi" "控制板类型"() -> (w300:string)
      n389 = global write "全局_配置.vi" "CAN打开标志"(FALSE ("CAN打开标志")) -> ()
      n390 = local write "加载配置文件列表"(u16 0) -> ()
      n391 = call "读写配置文件.vi"("文件名称"=w300, "m_bRead"=TRUE) -> ("BoardConfig_output"=w313:T3)  [unwired: 9 in]
      n392 = global write "试验配置信息.vi" "配置文件序号"(u16 0 ("配置文件序号")) -> ()
      n393 = Unbundle By Name(w313) -> ("数字量输入信号路数"=w307:i32, "数字量输出信号路数"=w306:i32, "DSP模拟量输入信号路数"=w305:u32, "DSP模拟量输入信号幅值"=w311:u32, "AD模拟量输入信号路数"=w304:u32, "AD模拟量输入信号幅值"=w308:u32, "RS232通信路数"=w303:u32, "RS232波特率"=w312:dbl, "RS485通信路数"=w302:u32, "CAN通信路数"=w301:i32)  [unwired: 7 out]
      n394 = global write "全局_配置.vi" "BoardConfig"(w313) -> ()
      n395 = case shown="0, 默认" w311 {
        tunnel: [3.3 10.0 24.0] -> w310
        frame 0, Default {
        }
        frame 1 {
        }
        frame 2 {
        }
      }
      n396 = case shown="2" w308 {
        tunnel: [6.0 10.0 24.0] -> w309
        frame 0, Default {
        }
        frame 1 {
        }
        frame 2 {
        }
      }
      n397 = global write "全局_配置.vi" "模拟量误差"(w312) -> ()
      n398 = global write "全局_配置.vi" "数字量输入路数"(w307) -> ()
      n399 = global write "全局_配置.vi" "数字量输出路数"(w306) -> ()
      n400 = global write "全局_配置.vi" "dsp模拟量输入路数"(w305) -> ()
      n401 = global write "全局_配置.vi" "ad模拟量输入路数"(w304) -> ()
      n402 = global write "试验配置信息.vi" "自测CAN路数"(w301) -> ()
      n403 = global write "全局_配置.vi" "R485路数"(w302) -> ()
      n404 = global write "全局_配置.vi" "CAN波特率"(u16 250 ("CAN波特率")) -> ()
      n405 = global write "全局_配置.vi" "R232路数"(w303) -> ()
      n406 = global write "全局_配置.vi" "DSP模拟量量程范围"(w310) -> ()
      n407 = global write "全局_配置.vi" "ARM模拟量量程范围"(w309) -> ()
      n408 = disable-structure shown="禁用" {
        frame Disabled {
          (unwired) "192.168.1.15" ("本机IP")
          (unwired) "192.168.1.10" ("控制板IP")
        }
        frame Enabled {
        }
      }
      n409 = global write "全局_配置.vi" "CAN发送帧数"(u32 100 ("CAN发送帧数")) -> ()
      n410 = global write "全局_配置.vi" "超时时间_10"(10.0 ("超时时间_102")) -> ()
      n411 = global write "全局_配置.vi" "超时时间_10"(5.0 ("超时时间_10")) -> ()
      n412 = global write "全局_配置.vi" "超时时间_2"(2.0 ("超时时间_2")) -> ()
      n413 = global write "全局_配置.vi" "控制板端口"(u16 6600 ("控制板端口")) -> ()
      n414 = global write "全局_配置.vi" "本机端口"(u16 6601 ("本机端口")) -> ()
      n415 = global write "全局_配置.vi" "本机IP"("192.168.1.15" ("本机IP")) -> ()
      n416 = global write "全局_配置.vi" "控制板IP"("192.168.1.10" ("控制板IP")) -> ()
    }
    frame #2 {
      w332 = 16 ("自测DI路数")
      n417 = global write "试验配置信息.vi" "自测类型3路数"(80 ("自测DI路数")) -> ()
      n418 = global write "试验配置信息.vi" "自测类型1路数"(w332) -> ()
      n419 = global write "试验配置信息.vi" "自测类型2路数"(w332) -> ()
      n420 = global write "试验配置信息.vi" "自测类型4路数"(w332) -> ()
      n421 = global write "试验配置信息.vi" "自测485路数"(1 ("自测485路数")) -> ()
      n422 = global write "试验配置信息.vi" "自测LAN路数"(1 ("自测LAN路数")) -> ()
    }
    frame #3 {
      w364 = TRUE ("单选_数字量输入")
      # "自动测试"
      n423 = case shown="0, 默认" 0 {
        tunnel: [cluster{u32, u32}[] [{1985280, 1985280}] cluster{u32, u32}[] [{61205, 6618880}] cluster{u32, u32}[] [{16730410, 16711680}]] -> w363
        frame 0, Default {
        }
        frame 1 {
        }
        frame 2 {
        }
      }
      n424 = property on="数字量输入检测" class="Bool (严格)"("Colors [4]"=w363) -> ()  [unwired: 2 in, 2 out]
      n425 = property on="数字量输出检测" class="Bool (严格)"("Colors [4]"=w363) -> ()  [unwired: 2 in, 2 out]
      n426 = property on="模拟量AD输入检测" class="Bool (严格)"("Colors [4]"=w363) -> ()  [unwired: 2 in, 2 out]
      n427 = property on="CAN总线检测" class="Bool (严格)"("Colors [4]"=w363) -> ()  [unwired: 2 in, 2 out]
      n428 = global write "自动测试结果.vi" "DI自动测试结果"(string[][] [["序号", "检测内容", "结果"]] ("自动测试结果")) -> ()
      n429 = property on="LAN总线检测" class="Bool (严格)"("Colors [4]"=w363) -> ()  [unwired: 2 in, 2 out]
      n430 = property on="RS232总线检测" class="Bool (严格)"("Colors [4]"=w363) -> ()  [unwired: 2 in, 2 out]
      n431 = property on="RS485总线检测" class="Bool (严格)"("Colors [4]"=w363) -> ()  [unwired: 2 in, 2 out]
      n432 = property on="模拟量DSP输入检测" class="Bool (严格)"("Colors [4]"=w363) -> ()  [unwired: 2 in, 2 out]
      n433 = property on="函数类型1检测" class="Bool (严格)"("Colors [4]"=w363) -> ()  [unwired: 2 in, 2 out]
      n434 = property on="函数类型2检测" class="Bool (严格)"("Colors [4]"=w363) -> ()  [unwired: 2 in, 2 out]
      n435 = property on="函数类型3检测" class="Bool (严格)"("Colors [4]"=w363) -> ()  [unwired: 2 in, 2 out]
      n436 = property on="函数类型4检测" class="Bool (严格)"("Colors [4]"=w363) -> ()  [unwired: 2 in, 2 out]
      n437 = global write "试验配置信息.vi" "自测类数"(0 ("自动测试个数")) -> ()
      n438 = local write "str_报告编号"("B001001000001" ("通知")) -> ()
      n439 = local write "str_测试地点"("1号实验室" ("str_测试地点")) -> ()
      n440 = global read "试验配置信息.vi" "自测类型1路数"() -> (w350:i32)
      n441 = global read "试验配置信息.vi" "自测类型1路数"() -> (w361:i32)
      n442 = global read "试验配置信息.vi" "自测类型2路数"() -> (w358:i32)
      n443 = global read "试验配置信息.vi" "自测类型3路数"() -> (w355:i32)
      n444 = global read "试验配置信息.vi" "自测类型4路数"() -> (w352:i32)
      n445 = Initialize Array(TRUE, 5 ("维数大小"), 16 ("维数大小")) -> (w340:bool[][])
      n446 = Initialize Array(TRUE, 5 ("维数大小"), 16 ("维数大小")) -> (w345:bool[][])
      n447 = Initialize Array(0.0, w350) -> (w349:dbl[])
      n448 = Initialize Array(TRUE ("元素"), w361) -> (w362:bool[])
      n449 = Initialize Array(TRUE ("元素"), w358) -> (w357:bool[])
      n450 = Initialize Array(TRUE ("元素"), w355) -> (w356:bool[])
      n451 = Initialize Array(TRUE ("元素"), w352) -> (w351:bool[])
      n452 = Initialize Array(TRUE ("元素"), 4 ("维数大小")) -> (w370:bool[])
      n453 = Initialize Array(TRUE ("元素"), 1 ("维数大小")) -> (w369:bool[])
      n454 = local write "单选_数字量输入"(w364) -> ()
      n455 = local write "单选_数字量输出"(w364) -> ()
      n456 = local write "单选_DSP输入"(w364) -> ()
      n457 = local write "单选_CAN检测"(w364) -> ()
      n458 = local write "单选_LAN检测"(w364) -> ()
      n459 = local write "单选_R232检测"(w364) -> ()
      n460 = local write "单选_R485检测"(w364) -> ()
      n461 = local write "单选_AD输入"(w364) -> ()
      n462 = Initialize Array(TRUE ("元素"), 16 ("维数大小")) -> (w377:bool[])
      n463 = Initialize Array(TRUE ("元素"), 2 ("维数大小")) -> (w366:bool[])
      n464 = Initialize Array(TRUE ("元素"), 16 ("维数大小")) -> (w372:bool[])
      n465 = global write "自动测试结果.vi" "Auto_DO_R"(w340) -> ()
      n466 = global write "自动测试结果.vi" "Auto_DI_R"(w345) -> ()
      n467 = global write "自动测试结果.vi" "Auto_func_1_max_WC"(w349) -> ()
      n468 = global write "自动测试结果.vi" "Auto_func_1_R"(w362) -> ()
      n469 = global write "自动测试结果.vi" "Auto_func_2_R"(w357) -> ()
      n470 = global write "自动测试结果.vi" "Auto_func_3_R"(w356) -> ()
      n471 = global write "自动测试结果.vi" "Auto_func_4_R"(w351) -> ()
      n472 = global write "自动测试结果.vi" "Auto_RS485_R"(w369) -> ()
      n473 = global write "自动测试结果.vi" "Auto_RS232_R"(w366) -> ()
      n474 = global write "自动测试结果.vi" "Auto_CAN_R"(w370) -> ()
      n475 = global write "自动测试结果.vi" "Auto_DSP_R"(w377) -> ()
      n476 = global write "自动测试结果.vi" "Auto_AD_R"(w372) -> ()
      n477 = local write "单选_函数类型1"(w364) -> ()
      n478 = local write "单选_函数类型2"(w364) -> ()
      n479 = local write "单选_函数类型3"(w364) -> ()
      n480 = local write "单选_函数类型4"(w364) -> ()
    }
    frame #4 {
      n481 = call "实验配置信息读取和写入.vi"("读取写入"=FALSE) -> ("输出簇"=w399:T1)  [unwired: 8 in]
      n482 = Unbundle By Name(w399) -> ("str_报告编号"=w397:string, "str_测试编号"=w396:string, "str_测试人员"=w394:string, "str_测试地点"=w395:string)
      n483 = Initialize Array(TRUE, 8 ("维数大小")) -> (w392:bool[])
      n484 = Initialize Array(TRUE, 4 ("维数大小")) -> (w389:bool[])
      n485 = call <vilib>:"RGB to Color.vi"("B"=255 ("维数大小"), "G"=0 ("维数大小"), "R"=0 ("维数大小")) -> ("Color"=w386:u32)
      n486 = global write "试验配置信息.vi" "板卡II自动检测结果"(w389) -> ()
      n487 = local write "str_报告编号"(w397) -> ()
      n488 = local write "str_测试编号"(w396) -> ()
      n489 = property on="进度提示" class="Str"("Text.TextColor"=w386) -> ()  [unwired: 2 in, 2 out]
      n490 = local write "进度提示"("测试准备就绪......") -> ()
      n491 = global write "试验配置信息.vi" "自动检测结果"(w392) -> ()
      n492 = local write "str_测试地点"(w395) -> ()
      n493 = local write "str_测试人员"(w394) -> ()
    }
  }
  n494 = Obtain Notifier(name (unnamed)=w10, notification data type=w10) -> (notifier out=w9:refnum<notifier>, error out=w8:errorcluster)  [unwired: 2 in, 1 out]
  n495 = while {
    tunnel: w9 -> [w409]
    tunnel: w8 -> [w408]
    tunnel: [w407] -> w7
    tunnel: [w406] -> w6
    stop <- w401 stop-if-true
    n496 = Wait Until Next ms Multiple(millisecond multiple=u32 20 ("毫秒倍数")) -> ()  [unwired: 1 out]
    n497 = Wait on Notification(notifier=w409, timeout in ms (-1)=20 ("超时毫秒(-1)"), error in (no error)=w408) -> (notifier out=w407:refnum<notifier>, notification=w404:string, error out=w406:errorcluster)  [unwired: 1 in, 1 out]
    n498 = Equal?(x=w404, y="Auto" ("通知")) -> (x = y?=w403:bool)
    n499 = case shown="真" w403 {
      frame False {
      }
      frame True {
        n500 = stacked-sequence {
          frame #0 {
            # "数字量输入"
            n501 = local read "单选_数字量输入"() -> (w410:bool)
            n502 = stacked-sequence {
              tunnel: w410 -> [w412 w413]
              frame #0 {
                n503 = call "数字量输入自动检测.vi"("选择?"=w412) -> ()  [unwired: 11 in]
                n504 = local write "进度提示"("正在进行数字量输入测试......") -> ()
              }
              frame #1 {
                n505 = case shown="真" w413 {
                  frame False {
                  }
                  frame True {
                    n506 = global read "试验配置信息.vi" "自动检测结果"() -> (w415:bool[])
                    n507 = Index Array(array=w415, index=0) -> (element=w417:bool)
                    n508 = case shown="真" w417 {
                      tunnel: [2 1] -> w418
                      frame False {
                      }
                      frame True {
                      }
                    }
                    n509 = case shown="0, 默认" w418 {
                      tunnel: [cluster{u32, u32}[] [{1985280, 1985280}] cluster{u32, u32}[] [{61205, 6618880}] cluster{u32, u32}[] [{16730410, 16711680}]] -> w414
                      frame 0, Default {
                      }
                      frame 1 {
                      }
                      frame 2 {
                      }
                    }
                    n510 = property on="数字量输入检测" class="Bool (严格)"("Colors [4]"=w414) -> ()  [unwired: 2 in, 2 out]
                  }
                }
              }
            }
          }
          frame #1 {
            # "数字量输出"
            n511 = local read "单选_数字量输出"() -> (w424:bool)
            n512 = stacked-sequence {
              tunnel: w424 -> [w426 w427]
              frame #0 {
                n513 = call "自动数量输出.vi"("选择？"=w426) -> ()  [unwired: 11 in]
                n514 = local write "进度提示"("正在进行数字量输出测试......") -> ()
              }
              frame #1 {
                n515 = case shown="真" w427 {
                  frame False {
                  }
                  frame True {
                    n516 = global read "试验配置信息.vi" "自动检测结果"() -> (w429:bool[])
                    n517 = Index Array(array=w429, index=1) -> (element=w431:bool)
                    n518 = case shown="假" w431 {
                      tunnel: [2 1] -> w432
                      frame False {
                      }
                      frame True {
                      }
                    }
                    n519 = case shown="0, 默认" w432 {
                      tunnel: [cluster{u32, u32}[] [{1985280, 1985280}] cluster{u32, u32}[] [{61205, 6618880}] cluster{u32, u32}[] [{16730410, 16711680}]] -> w428
                      frame 0, Default {
                      }
                      frame 1 {
                      }
                      frame 2 {
                      }
                    }
                    n520 = property on="数字量输出检测" class="Bool (严格)"("Colors [4]"=w428) -> ()  [unwired: 2 in, 2 out]
                  }
                }
              }
            }
          }
          frame #2 {
            # "模拟量输入"
            n521 = local read "单选_DSP输入"() -> (w439:bool)
            n522 = property on="单选_AD输入" class="Bool (严格)"() -> ("Value"=w438:bool)  [unwired: 2 in, 2 out]
            n523 = stacked-sequence {
              tunnel: w439 -> [w442 w444]
              tunnel: w438 -> [w441 w443]
              frame #0 {
                n524 = call "模拟量输入自动测试.vi"("AD选择?"=w441, "DSP选择?"=w442) -> ()  [unwired: 10 in]
                n525 = local write "进度提示"("正在进行模拟量测试......") -> ()
              }
              frame #1 {
                n526 = stacked-sequence {
                  tunnel: w444 -> [w445 _]
                  tunnel: w443 -> [_ w456]
                  frame #0 {
                    n527 = case shown="真" w445 {
                      frame False {
                      }
                      frame True {
                        n528 = global read "试验配置信息.vi" "自动检测结果"() -> (w447:bool[])
                        n529 = Index Array(array=w447, index=2) -> (element=w449:bool)
                        n530 = case shown="假" w449 {
                          tunnel: [2 1] -> w450
                          frame False {
                          }
                          frame True {
                          }
                        }
                        n531 = case shown="0, 默认" w450 {
                          tunnel: [cluster{u32, u32}[] [{1985280, 1985280}] cluster{u32, u32}[] [{61205, 6618880}] cluster{u32, u32}[] [{16730410, 16711680}]] -> w446
                          frame 0, Default {
                          }
                          frame 1 {
                          }
                          frame 2 {
                          }
                        }
                        n532 = property on="模拟量DSP输入检测" class="Bool (严格)"("Colors [4]"=w446) -> ()  [unwired: 2 in, 2 out]
                      }
                    }
                  }
                  frame #1 {
                    n533 = case shown="真" w456 {
                      frame False {
                      }
                      frame True {
                        n534 = global read "试验配置信息.vi" "自动检测结果"() -> (w458:bool[])
                        n535 = Index Array(array=w458, index=3) -> (element=w460:bool)
                        n536 = case shown="假" w460 {
                          tunnel: [2 1] -> w461
                          frame False {
                          }
                          frame True {
                          }
                        }
                        n537 = case shown="0, 默认" w461 {
                          tunnel: [cluster{u32, u32}[] [{1985280, 1985280}] cluster{u32, u32}[] [{61205, 6618880}] cluster{u32, u32}[] [{16730410, 16711680}]] -> w457
                          frame 0, Default {
                          }
                          frame 1 {
                          }
                          frame 2 {
                          }
                        }
                        n538 = property on="模拟量AD输入检测" class="Bool (严格)"("Colors [4]"=w457) -> ()  [unwired: 2 in, 2 out]
                      }
                    }
                  }
                }
              }
            }
          }
          frame #3 {
            # "串口"
            n539 = local read "单选_R232检测"() -> (w468:bool)
            n540 = local read "单选_R485检测"() -> (w467:bool)
            n541 = stacked-sequence {
              tunnel: w468 -> [w471 w473]
              tunnel: w467 -> [w470 w472]
              frame #0 {
                n542 = call "串口自动测试.vi"("RS485选择"=w470, "RS232选择"=w471) -> ()  [unwired: 10 in]
                n543 = local write "进度提示"("正在进行串口测试......") -> ()
              }
              frame #1 {
                n544 = stacked-sequence {
                  tunnel: w473 -> [w474 _]
                  tunnel: w472 -> [_ w485]
                  frame #0 {
                    n545 = case shown="真" w474 {
                      frame False {
                      }
                      frame True {
                        n546 = global read "试验配置信息.vi" "自动检测结果"() -> (w476:bool[])
                        n547 = Index Array(array=w476, index=4) -> (element=w478:bool)
                        n548 = case shown="假" w478 {
                          tunnel: [2 1] -> w479
                          frame False {
                          }
                          frame True {
                          }
                        }
                        n549 = case shown="0, 默认" w479 {
                          tunnel: [cluster{u32, u32}[] [{1985280, 1985280}] cluster{u32, u32}[] [{61205, 6618880}] cluster{u32, u32}[] [{16730410, 16711680}]] -> w475
                          frame 0, Default {
                          }
                          frame 1 {
                          }
                          frame 2 {
                          }
                        }
                        n550 = property on="RS232总线检测" class="Bool (严格)"("Colors [4]"=w475) -> ()  [unwired: 2 in, 2 out]
                      }
                    }
                  }
                  frame #1 {
                    n551 = case shown="真" w485 {
                      frame False {
                      }
                      frame True {
                        n552 = global read "试验配置信息.vi" "自动检测结果"() -> (w487:bool[])
                        n553 = Index Array(array=w487, index=5) -> (element=w489:bool)
                        n554 = case shown="假" w489 {
                          tunnel: [2 1] -> w490
                          frame False {
                          }
                          frame True {
                          }
                        }
                        n555 = case shown="0, 默认" w490 {
                          tunnel: [cluster{u32, u32}[] [{1985280, 1985280}] cluster{u32, u32}[] [{61205, 6618880}] cluster{u32, u32}[] [{16730410, 16711680}]] -> w486
                          frame 0, Default {
                          }
                          frame 1 {
                          }
                          frame 2 {
                          }
                        }
                        n556 = property on="RS485总线检测" class="Bool (严格)"("Colors [4]"=w486) -> ()  [unwired: 2 in, 2 out]
                      }
                    }
                  }
                }
              }
            }
          }
          frame #4 {
            # "CAN"
            n557 = local read "单选_CAN检测"() -> (w496:bool)
            n558 = stacked-sequence {
              tunnel: w496 -> [w498 w499]
              frame #0 {
                n559 = call "CAN自动测试.vi"("选择?"=w498) -> ()  [unwired: 11 in]
                n560 = local write "进度提示"("正在进行CAN测试......") -> ()
              }
              frame #1 {
                n561 = case shown="真" w499 {
                  frame False {
                  }
                  frame True {
                    n562 = global read "试验配置信息.vi" "自动检测结果"() -> (w501:bool[])
                    n563 = Index Array(array=w501, index=6) -> (element=w503:bool)
                    n564 = case shown="假" w503 {
                      tunnel: [2 1] -> w504
                      frame False {
                      }
                      frame True {
                      }
                    }
                    n565 = case shown="0, 默认" w504 {
                      tunnel: [cluster{u32, u32}[] [{1985280, 1985280}] cluster{u32, u32}[] [{61205, 6618880}] cluster{u32, u32}[] [{16730410, 16711680}]] -> w500
                      frame 0, Default {
                      }
                      frame 1 {
                      }
                      frame 2 {
                      }
                    }
                    n566 = property on="CAN总线检测" class="Bool (严格)"("Colors [4]"=w500) -> ()  [unwired: 2 in, 2 out]
                  }
                }
              }
            }
          }
          frame #5 {
            # "以太网"
            n567 = local read "单选_LAN检测"() -> (w510:bool)
            n568 = stacked-sequence {
              tunnel: w510 -> [w512 w513]
              frame #0 {
                n569 = call "以太网自动测试.vi"("选择?"=w512) -> ()  [unwired: 11 in]
                n570 = local write "进度提示"("正在进行LAN测试......") -> ()
              }
              frame #1 {
                n571 = case shown="真" w513 {
                  frame False {
                  }
                  frame True {
                    n572 = global read "试验配置信息.vi" "自动检测结果"() -> (w515:bool[])
                    n573 = Index Array(array=w515, index=7) -> (element=w517:bool)
                    n574 = case shown="假" w517 {
                      tunnel: [2 1] -> w518
                      frame False {
                      }
                      frame True {
                      }
                    }
                    n575 = case shown="0, 默认" w518 {
                      tunnel: [cluster{u32, u32}[] [{1985280, 1985280}] cluster{u32, u32}[] [{61205, 6618880}] cluster{u32, u32}[] [{16730410, 16711680}]] -> w514
                      frame 0, Default {
                      }
                      frame 1 {
                      }
                      frame 2 {
                      }
                    }
                    n576 = property on="LAN总线检测" class="Bool (严格)"("Colors [4]"=w514) -> ()  [unwired: 2 in, 2 out]
                  }
                }
              }
            }
          }
          frame #6 {
            # "统计合格率"
            n577 = call "统计合格率.vi"() -> ()  [unwired: 12 in]
          }
          frame #7 {
            n578 = flat-sequence {
              frame #0 {
                # "报告存储"
                n579 = Get Date/Time In Seconds() -> (seconds since 1Jan1904=w524:timestamp)
                n580 = call "报告存储.vi"("试验时间"=w524) -> ()  [unwired: 11 in]
              }
              frame #1 {
                n581 = call "完成"() -> ()  [unwired: 10 in, 2 out]
              }
            }
            n582 = disable-structure shown="禁用" {
              frame Disabled {
                n583 = Get Date/Time In Seconds() -> (seconds since 1Jan1904=w525:timestamp)
                n584 = call "测试报告摘要4.vi"("打印?"=FALSE, "试验时间"=w525) -> ()  [unwired: 10 in]
              }
              frame Enabled {
              }
            }
          }
          frame #8 {
            w528 = T2."Enabled" ("禁用")
            n585 = case shown="0, 默认" 0 {
              tunnel: [cluster{u32, u32}[] [{1985280, 1985280}] cluster{u32, u32}[] [{61205, 6618880}] cluster{u32, u32}[] [{16730410, 16711680}]] -> w529
              frame 0, Default {
              }
              frame 1 {
              }
              frame 2 {
              }
            }
            n586 = property on="数字量输入检测" class="Bool (严格)"("Colors [4]"=w529) -> ()  [unwired: 2 in, 2 out]
            n587 = property on="数字量输出检测" class="Bool (严格)"("Colors [4]"=w529) -> ()  [unwired: 2 in, 2 out]
            n588 = property on="模拟量AD输入检测" class="Bool (严格)"("Colors [4]"=w529) -> ()  [unwired: 2 in, 2 out]
            n589 = property on="CAN总线检测" class="Bool (严格)"("Colors [4]"=w529) -> ()  [unwired: 2 in, 2 out]
            n590 = local write "进度提示"("测试完毕......") -> ()
            n591 = property on="LAN总线检测" class="Bool (严格)"("Colors [4]"=w529) -> ()  [unwired: 2 in, 2 out]
            n592 = property on="RS232总线检测" class="Bool (严格)"("Colors [4]"=w529) -> ()  [unwired: 2 in, 2 out]
            n593 = property on="RS485总线检测" class="Bool (严格)"("Colors [4]"=w529) -> ()  [unwired: 2 in, 2 out]
            n594 = property on="模拟量DSP输入检测" class="Bool (严格)"("Colors [4]"=w529) -> ()  [unwired: 2 in, 2 out]
            n595 = property on="btn_数字输入" class="Bool"("DisabledEnum"=w528) -> ()  [unwired: 2 in, 2 out]
            n596 = property on="btn_数字输出" class="Bool"("DisabledEnum"=w528) -> ()  [unwired: 2 in, 2 out]
            n597 = property on="btn_DSP输入" class="Bool"("DisabledEnum"=w528) -> ()  [unwired: 2 in, 2 out]
            n598 = property on="btn_CAN总线" class="Bool"("DisabledEnum"=w528) -> ()  [unwired: 2 in, 2 out]
            n599 = property on="btn_R232_485总线" class="Bool"("DisabledEnum"=w528) -> ()  [unwired: 2 in, 2 out]
            n600 = property on="btn_LAN总线" class="Bool"("DisabledEnum"=w528) -> ()  [unwired: 2 in, 2 out]
            n601 = property on="btn_自动开始检测类型2" class="Bool"("DisabledEnum"=w528) -> ()  [unwired: 2 in, 2 out]
            n602 = property on="函数类型 1" class="Bool"("DisabledEnum"=w528) -> ()  [unwired: 2 in, 2 out]
            n603 = property on="函数类型 2" class="Bool"("DisabledEnum"=w528) -> ()  [unwired: 2 in, 2 out]
            n604 = property on="函数类型 3" class="Bool"("DisabledEnum"=w528) -> ()  [unwired: 2 in, 2 out]
            n605 = property on="函数类型 4" class="Bool"("DisabledEnum"=w528) -> ()  [unwired: 2 in, 2 out]
          }
        }
      }
    }
    n606 = local read "退出？"() -> (w401:bool)
  }
  n607 = Obtain Notifier(name (unnamed)=w5, notification data type=w5) -> (notifier out=w4:refnum<notifier>, error out=w3:errorcluster)  [unwired: 2 in, 1 out]
  n608 = while {
    tunnel: w4 -> [w543]
    tunnel: w3 -> [w542]
    tunnel: [w541] -> w2
    tunnel: [w540] -> w1
    stop <- w534 stop-if-true
    n609 = Wait Until Next ms Multiple(millisecond multiple=u32 20 ("毫秒倍数")) -> ()  [unwired: 1 out]
    n610 = Wait on Notification(notifier=w543, timeout in ms (-1)=20 ("超时毫秒(-1)"), error in (no error)=w542) -> (notifier out=w541:refnum<notifier>, notification=w538:string, error out=w540:errorcluster)  [unwired: 1 in, 1 out]
    n611 = Equal?(x=w538, y="Auto_2" ("通知")) -> (x = y?=w535:bool)
    n612 = case shown="真" w535 {
      frame False {
      }
      frame True {
        n613 = stacked-sequence {
          frame #0 {
            # "类型1测试"
            n614 = local read "单选_函数类型1"() -> (w544:bool)
            n615 = case shown="真" w544 {
              frame False {
              }
              frame True {
                n616 = stacked-sequence {
                  frame #0 {
                    n617 = stacked-sequence {
                      frame #0 {
                        n618 = call "测试类型1自动测试一组.vi"() -> ()  [unwired: 10 in]
                      }
                      frame #1 {
                        n619 = call "自动测试类型1统计结果.vi"() -> ()  [unwired: 12 in]
                      }
                    }
                    n620 = local write "进度提示"("正在进行类型1测试......") -> ()
                  }
                  frame #1 {
                    n621 = global read "试验配置信息.vi" "板卡II自动检测结果"() -> (w549:bool[])
                    n622 = Index Array(array=w549, index=0) -> (element=w547:bool)
                    n623 = case shown="假" w547 {
                      tunnel: [2 1] -> w546
                      frame False {
                      }
                      frame True {
                      }
                    }
                    n624 = case shown="0, 默认" w546 {
                      tunnel: [cluster{u32, u32}[] [{1985280, 1985280}] cluster{u32, u32}[] [{61205, 6618880}] cluster{u32, u32}[] [{16730410, 16711680}]] -> w550
                      frame 0, Default {
                      }
                      frame 1 {
                      }
                      frame 2 {
                      }
                    }
                    n625 = property on="函数类型1检测" class="Bool (严格)"("Colors [4]"=w550) -> ()  [unwired: 2 in, 2 out]
                  }
                }
              }
            }
          }
          frame #1 {
            # "类型2测试"
            n626 = stacked-sequence {
              frame #0 {
                n627 = local write "进度提示"("正在进行类型2测试......") -> ()
              }
              frame #1 {
                n628 = global read "试验配置信息.vi" "板卡II自动检测结果"() -> (w560:bool[])
                n629 = Index Array(array=w560, index=1) -> (element=w558:bool)
                n630 = case shown="假" w558 {
                  tunnel: [2 1] -> w557
                  frame False {
                  }
                  frame True {
                  }
                }
                n631 = case shown="0, 默认" w557 {
                  tunnel: [cluster{u32, u32}[] [{1985280, 1985280}] cluster{u32, u32}[] [{61205, 6618880}] cluster{u32, u32}[] [{16730410, 16711680}]] -> w561
                  frame 0, Default {
                  }
                  frame 1 {
                  }
                  frame 2 {
                  }
                }
                n632 = property on="函数类型2检测" class="Bool (严格)"("Colors [4]"=w561) -> ()  [unwired: 2 in, 2 out]
              }
            }
          }
          frame #2 {
            # "类型3测试"
            n633 = local read "单选_函数类型3"() -> (w567:bool)
            n634 = stacked-sequence {
              tunnel: w567 -> [w569 _]
              frame #0 {
                n635 = call "类型3自动测试.vi"("选择?"=w569) -> ()  [unwired: 11 in]
                n636 = local write "进度提示"("正在进行类型3测试......") -> ()
              }
              frame #1 {
                n637 = global read "试验配置信息.vi" "板卡II自动检测结果"() -> (w573:bool[])
                n638 = Index Array(array=w573, index=2) -> (element=w571:bool)
                n639 = case shown="假" w571 {
                  tunnel: [2 1] -> w570
                  frame False {
                  }
                  frame True {
                  }
                }
                n640 = case shown="0, 默认" w570 {
                  tunnel: [cluster{u32, u32}[] [{1985280, 1985280}] cluster{u32, u32}[] [{61205, 6618880}] cluster{u32, u32}[] [{16730410, 16711680}]] -> w574
                  frame 0, Default {
                  }
                  frame 1 {
                  }
                  frame 2 {
                  }
                }
                n641 = property on="函数类型3检测" class="Bool (严格)"("Colors [4]"=w574) -> ()  [unwired: 2 in, 2 out]
              }
            }
          }
          frame #3 {
            # "类型4测试"
            n642 = stacked-sequence {
              frame #0 {
                n643 = local write "进度提示"("正在进行类型4测试......") -> ()
              }
              frame #1 {
                n644 = global read "试验配置信息.vi" "板卡II自动检测结果"() -> (w584:bool[])
                n645 = Index Array(array=w584, index=3) -> (element=w582:bool)
                n646 = case shown="假" w582 {
                  tunnel: [2 1] -> w581
                  frame False {
                  }
                  frame True {
                  }
                }
                n647 = case shown="0, 默认" w581 {
                  tunnel: [cluster{u32, u32}[] [{1985280, 1985280}] cluster{u32, u32}[] [{61205, 6618880}] cluster{u32, u32}[] [{16730410, 16711680}]] -> w585
                  frame 0, Default {
                  }
                  frame 1 {
                  }
                  frame 2 {
                  }
                }
                n648 = property on="函数类型4检测" class="Bool (严格)"("Colors [4]"=w585) -> ()  [unwired: 2 in, 2 out]
              }
            }
          }
          frame #4 {
            # "统计合格率"
            n649 = call "二型板自动测试合格率统计.vi"() -> ()  [unwired: 12 in]
          }
          frame #5 {
            # "报告存储"
            n650 = flat-sequence {
              frame #0 {
                n651 = Get Date/Time In Seconds() -> (seconds since 1Jan1904=w591:timestamp)
                n652 = call "二型板测试报告存储.vi"("试验时间"=w591) -> ()  [unwired: 11 in]
              }
              frame #1 {
                n653 = call "完成2"() -> ()  [unwired: 10 in, 2 out]
              }
            }
          }
          frame #6 {
            w593 = T2."Enabled" ("禁用")
            n654 = case shown="0, 默认" 0 {
              tunnel: [cluster{u32, u32}[] [{1985280, 1985280}] cluster{u32, u32}[] [{61205, 6618880}] cluster{u32, u32}[] [{16730410, 16711680}]] -> w595
              frame 0, Default {
              }
              frame 1 {
              }
              frame 2 {
              }
            }
            n655 = property on="函数类型1检测" class="Bool (严格)"("Colors [4]"=w595) -> ()  [unwired: 2 in, 2 out]
            n656 = property on="函数类型2检测" class="Bool (严格)"("Colors [4]"=w595) -> ()  [unwired: 2 in, 2 out]
            n657 = property on="函数类型3检测" class="Bool (严格)"("Colors [4]"=w595) -> ()  [unwired: 2 in, 2 out]
            n658 = property on="函数类型4检测" class="Bool (严格)"("Colors [4]"=w595) -> ()  [unwired: 2 in, 2 out]
            n659 = local write "进度提示"("测试完毕......") -> ()
            n660 = property on="btn_数字输入" class="Bool"("DisabledEnum"=w593) -> ()  [unwired: 2 in, 2 out]
            n661 = property on="btn_数字输出" class="Bool"("DisabledEnum"=w593) -> ()  [unwired: 2 in, 2 out]
            n662 = property on="btn_DSP输入" class="Bool"("DisabledEnum"=w593) -> ()  [unwired: 2 in, 2 out]
            n663 = property on="btn_CAN总线" class="Bool"("DisabledEnum"=w593) -> ()  [unwired: 2 in, 2 out]
            n664 = property on="btn_R232_485总线" class="Bool"("DisabledEnum"=w593) -> ()  [unwired: 2 in, 2 out]
            n665 = property on="btn_LAN总线" class="Bool"("DisabledEnum"=w593) -> ()  [unwired: 2 in, 2 out]
            n666 = property on="函数类型 1" class="Bool"("DisabledEnum"=w593) -> ()  [unwired: 2 in, 2 out]
            n667 = property on="函数类型 2" class="Bool"("DisabledEnum"=w593) -> ()  [unwired: 2 in, 2 out]
            n668 = property on="函数类型 3" class="Bool"("DisabledEnum"=w593) -> ()  [unwired: 2 in, 2 out]
            n669 = property on="函数类型 4" class="Bool"("DisabledEnum"=w593) -> ()  [unwired: 2 in, 2 out]
            n670 = property on="btn_开始检测" class="Bool"("DisabledEnum"=w593) -> ()  [unwired: 2 in, 2 out]
          }
        }
      }
    }
    n671 = local read "退出？"() -> (w534:bool)
  }
  n672 = Release Notifier(notifier=w7, error in (no error)=w6) -> ()  [unwired: 1 in, 3 out]
  n673 = Release Notifier(notifier=w2, error in (no error)=w1) -> ()  [unwired: 1 in, 3 out]
